vi "ni579x Construct Command Set Attenuation.vi"(0 "Register Bus":T3, 1 "scope":string, 5 "attenuation [dB]":dbl format="%#_6p", 11 "Error In":errorcluster) -> (4 "Register Bus (out)":T3, 6 "User Command":T1 {"User Command ID" items=["Set Clock Select"=0, "Set CLK OUT Source"=1, "DAC Sync User Start"=2, "DAC Sync User End"=3, "Enable Baseband Amp"=5, "Set Rx Attenuation Pre-LNA"=7, "Set Rx Attenuation Post-LNA"=8, "Set Tx Attenuation"=9, "Set LO Filter"=32, "Set Front End Filter"=33, "Enable LO"=34, "Set Routing Mux"=37, "Read Current Rev Lower"=240, "Read Current Rev Upper"=241, "Read Oldest Compat Rev Lower"=242, "Read Oldest Compat Rev Upper"=243, "Re-Initialize"=255]; "User Data 1" format="%x"; "User Data 0" format="%x"}, 15 "Error Out":errorcluster)   [LabVIEW 2015, in "ni579x Config v2 Host.lvlib"]
uses:
  <instrlib>/ni579x/Config/v2/Host/ni579x Config v2 Host.lvlib
  <instrlib>/_niInstr/Register Bus/v0/Host/Public/Register Bus Session.ctl
  <instrlib>/_niInstr/Register Bus/v0/Host/Private/Session Data.ctl
  <instrlib>/ni579x/Config/v2/Shared/Types/ni579x User Command.ctl
  <instrlib>/ni579x/Config/v2/Shared/Types/ni579x User Command ID.ctl
  <instrlib>/ni579x/Config/v2/Shared/ni579x Config v2 Shared.lvlib
  <instrlib>/_niInstr/Register Bus/v0/Host/niInstr Register Bus v0 Host.lvlib
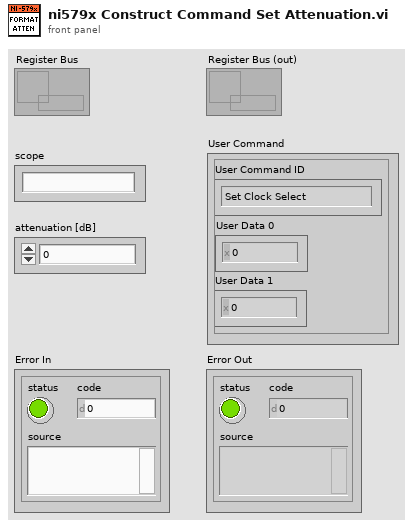
[diagram p1: front panel]
types:
  T1 = typedef "ni579x Config v2 Shared.lvlib/ni579x User Command.ctl" = cluster{"User Data 0":u8, "User Data 1":u8, "User Command ID":T2}
  T2 = typedef "ni579x Config v2 Shared.lvlib/ni579x User Command ID.ctl" = u8
  T3 = typedef "niInstr Register Bus v0 Host.lvlib/Register Bus Session.ctl" = refnum<queue>
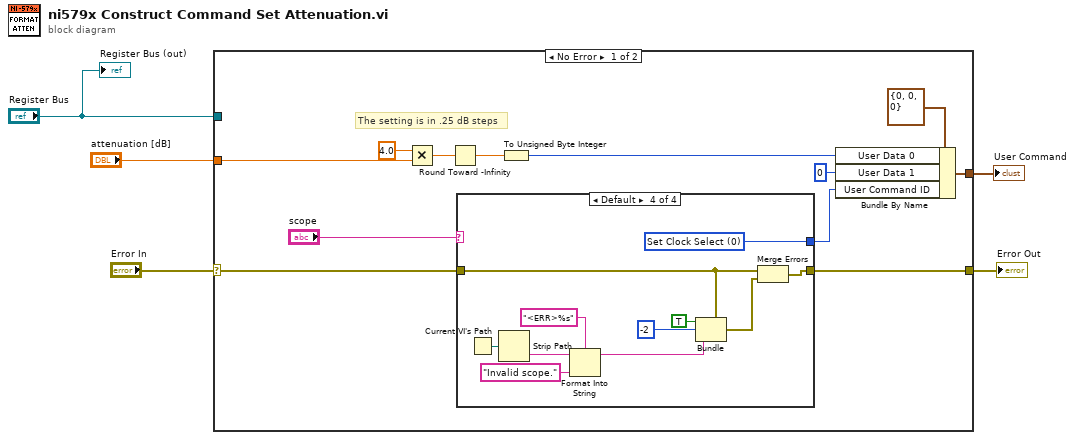
[diagram p0: block diagram]
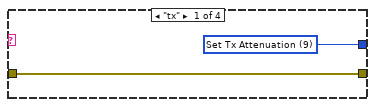
[diagram p2: hidden frame]
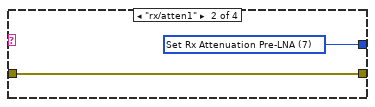
[diagram p3: hidden frame]
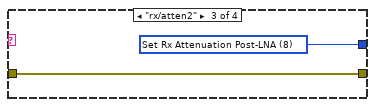
[diagram p4: hidden frame]
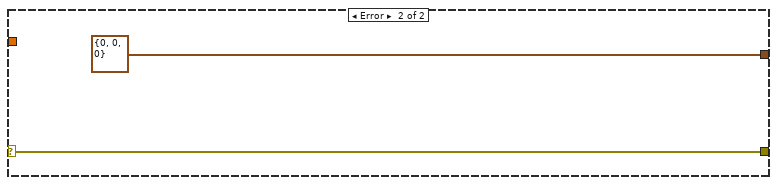
[diagram p5: hidden frame]
diagram:
  n1 = case shown="No Error" "Error In" {
    selector: "Error In" -> [w17 w36]
    tunnel: [w16 w36] -> w4
    tunnel: "Register Bus" -> [_ _]
    tunnel: "attenuation [dB]" -> [w9 _]
    tunnel: [w13 T1 {"User Data 0"=0, "User Data 1"=0, "User Command ID"=0} ("User Command")] -> w1
    frame No Error {
      # "The setting is in .25 dB steps"
      n2 = Multiply(x=4.0, y=w9) -> (x*y=w8:dbl)
      n3 = Round Toward -Infinity(1:w8) -> (0:w6:dbl)
      n4 = case shown="Default" "scope" {
        tunnel: w17 -> [w19 w21 w23 w30]
        tunnel: [w19 w21 w23 w25] -> w16
        tunnel: [w18 w20 w22 w24] -> w11
        frame "tx" {
          w18 = T2 9 items=["Set Clock Select"=0, "Set CLK OUT Source"=1, "DAC Sync User Start"=2, "DAC Sync User End"=3, "Enable Baseband Amp"=5, "Set Rx Attenuation Pre-LNA"=7, "Set Rx Attenuation Post-LNA"=8, "Set Tx Attenuation"=9, "Set LO Filter"=32, "Set Front End Filter"=33, "Enable LO"=34, "Set Routing Mux"=37, "Read Current Rev Lower"=240, "Read Current Rev Upper"=241, "Read Oldest Compat Rev Lower"=242, "Read Oldest Compat Rev Upper"=243, "Re-Initialize"=255] ("User Command ID")
        }
        frame "rx/atten1" {
          w20 = T2 7 items=["Set Clock Select"=0, "Set CLK OUT Source"=1, "DAC Sync User Start"=2, "DAC Sync User End"=3, "Enable Baseband Amp"=5, "Set Rx Attenuation Pre-LNA"=7, "Set Rx Attenuation Post-LNA"=8, "Set Tx Attenuation"=9, "Set LO Filter"=32, "Set Front End Filter"=33, "Enable LO"=34, "Set Routing Mux"=37, "Read Current Rev Lower"=240, "Read Current Rev Upper"=241, "Read Oldest Compat Rev Lower"=242, "Read Oldest Compat Rev Upper"=243, "Re-Initialize"=255] ("User Command ID")
        }
        frame "rx/atten2" {
          w22 = T2 8 items=["Set Clock Select"=0, "Set CLK OUT Source"=1, "DAC Sync User Start"=2, "DAC Sync User End"=3, "Enable Baseband Amp"=5, "Set Rx Attenuation Pre-LNA"=7, "Set Rx Attenuation Post-LNA"=8, "Set Tx Attenuation"=9, "Set LO Filter"=32, "Set Front End Filter"=33, "Enable LO"=34, "Set Routing Mux"=37, "Read Current Rev Lower"=240, "Read Current Rev Upper"=241, "Read Oldest Compat Rev Lower"=242, "Read Oldest Compat Rev Upper"=243, "Re-Initialize"=255] ("User Command ID")
        }
        frame Default {
          w24 = T2 0 items=["Set Clock Select"=0, "Set CLK OUT Source"=1, "DAC Sync User Start"=2, "DAC Sync User End"=3, "Enable Baseband Amp"=5, "Set Rx Attenuation Pre-LNA"=7, "Set Rx Attenuation Post-LNA"=8, "Set Tx Attenuation"=9, "Set LO Filter"=32, "Set Front End Filter"=33, "Enable LO"=34, "Set Routing Mux"=37, "Read Current Rev Lower"=240, "Read Current Rev Upper"=241, "Read Oldest Compat Rev Lower"=242, "Read Oldest Compat Rev Upper"=243, "Re-Initialize"=255] ("User Command ID")
          n5 = Current VI's Path() -> (path=w33:path)
          n6 = Strip Path(path=w33) -> (name=w32:string)  [unwired: 1 out]
          n7 = Format Into String(format string="<ERR>%s", initial string=w32, "Invalid scope." ("input 1")) -> (resulting string=w31:string)  [unwired: 1 in, 1 out]
          n8 = Bundle(cluster=w30, "status"=TRUE, "code"=-2, "source"=w31) -> (w29:errorcluster)
          n9 = Merge Errors(w30, w29) -> (w25:errorcluster)
        }
      }
      n10 = To Unsigned Byte Integer(number=w6) -> (unsigned 8bit integer=w7:u8)
      n11 = Bundle By Name(cluster=T1 {"User Data 0"=0, "User Data 1"=0, "User Command ID"=0} ("User Command"), "User Data 0"=w7, "User Data 1"=u8 0, "User Command ID"=w11) -> (w13:T1)
    }
    frame Error {
    }
  }
  "Error Out" <- w4
  "User Command" <- w1
  "Register Bus (out)" <- "Register Bus"
